vi "HRR-EloMecTester.vi"() -> ()   [LabVIEW 2019]
uses:
  <vilib>/FPGAPlugInAG/myRIO-1900/niLvFpga_Open_myRIO-1900.vi
  <vilib>/rvi/interface/common/dynamic/niFpgaDynamicAddResources.vi
  <vilib>/myRIO/Common/Instrument Driver Framework/Utilities/vis/FPGA Ref Manager.vi
  <vilib>/Utility/error.llb/Error Cluster From Error Code.vi
  <vilib>/myRIO/Common/Instrument Driver Framework/Utilities/vis/Ref Counter.vi
  <vilib>/rvi/interface/common/niFpgaWaitOnOcc.vi
  <vilib>/rvi/interface/nirviOpenFPGA/nirviOpenFPGA.xnode
  FPGA Bitfiles/MyRIOFPGATest_FPGATarget_FPGAMainDefault_pJ5Q7Xj1Ujo.lvbitx
  FPGA Main Default.vi
  <vilib>/rvi/interface/nirviMethod/nirviMethod.xnode
  <vilib>/FPGAPlugInAG/Dynamic/niLvFpga_ConfigureFifo_Dynamic.vi
  <vilib>/rvi/errors/niLvFpgaMergeErrorWithErrorCode.vi
  <vilib>/myRIO/Instrument Drivers/Utilities/Utilities.lvlib
panel:
  in  "stop":bool
  out "error out":errorcluster
  in  "Pos, Vel":u16[][](array[numeric])=[[660, 128], [360, 128], [360, 128], [670, 128], [370, 128], [670, 128], [670, 128], [360, 128]] max=1023 step=10
  out "Actual Depth":u32
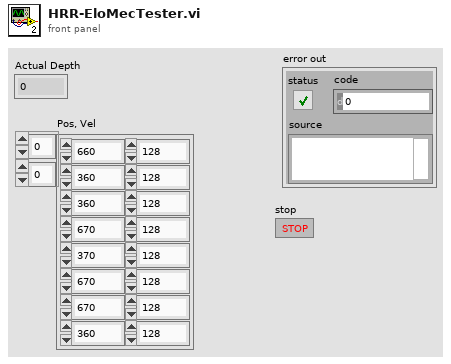
[diagram p1: front panel]
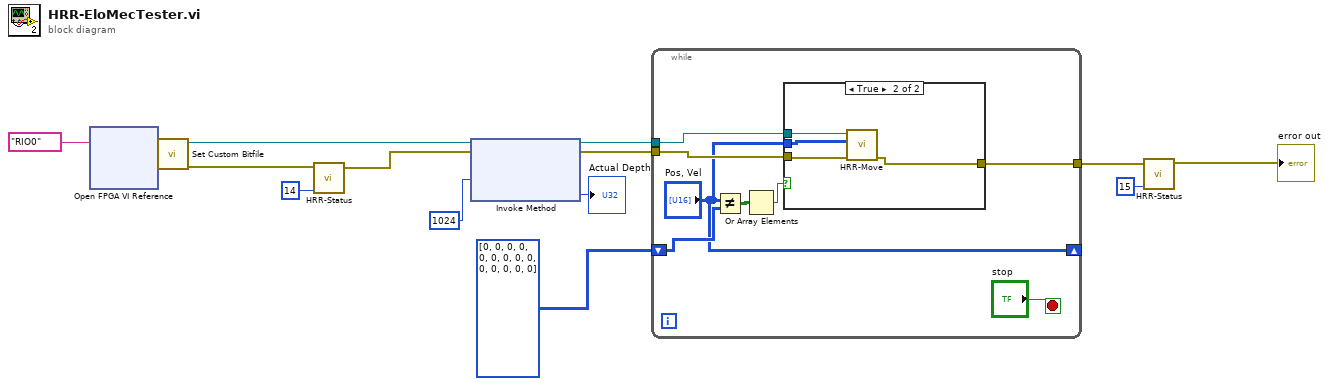
[diagram p0: block diagram]
diagram:
  n1 = xnode "Open FPGA VI Reference"("resource name"=tag "RIO0") -> ("FPGA VI Reference Out"=w13:refnum<k20>, "error out"=w14:errorcluster)  [unwired: 1 in]
  n2 = call <vilib>:"Set Custom Bitfile.vi"("error in (no error)"=w14, "Custom FPGA Reference In"=w13) -> ("error out"=w8:errorcluster, "Custom FPGA Reference Out"=w7:refnum<k20>)  [unwired: 8 in]
  n3 = call "HRR-Status.vi"("Status (U4)"=u8 14 ("number"), "error in (no error)"=w8) -> ("error out"=w10:errorcluster)  [unwired: 9 in]
  n4 = xnode "Invoke Method"("FPGA VI Reference In"=w7, "error in"=w10, "Requested Depth"=u32 1024) -> ("FPGA VI Reference Out"=w5:refnum<k20>, "error out"=w6:errorcluster, "Actual Depth"=→"Actual Depth":u32)
  n5 = while {
    tunnel: w6 -> [w23]
    tunnel: w5 -> [w22]
    tunnel: [w21] -> w3
    shift-right: ["Pos, Vel"] -> _
    shift-left: u16[][] [[0, 0], [0, 0], [0, 0], [0, 0], [0, 0], [0, 0], [0, 0]] ("Pos, Vel") -> [w19]
    stop <- "stop" stop-if-true
    n6 = Not Equal?(x="Pos, Vel", y=w19) -> (x != y?=w17:bool[][])
    n7 = Or Array Elements(Boolean array=w17) -> (logical OR=w18:bool)
    n8 = case shown="True" w18 {
      tunnel: w23 -> [w24 w28]
      tunnel: w22 -> [_ w27]
      tunnel: [w24 w26] -> w21
      tunnel: "Pos, Vel" -> [_ w25]
      frame False {
      }
      frame True {
        n9 = call "HRR-Move.vi"("error in"=w28, "Pos, Vel"=w25, "FPGA VI Reference In"=w27) -> ("error out"=w26:errorcluster)  [unwired: 7 in, 1 out]
      }
    }
  }
  n10 = call "HRR-Status.vi"("Status (U4)"=u8 15, "error in (no error)"=w3) -> ("error out"=→"error out":errorcluster)  [unwired: 9 in]
